vi "LogInfo2txt.vi"(7 "File ID":string, 11 "text":string) -> ()   [LabVIEW 2023, in "LoggingProber.lvlib"]
uses:
  LoggingProber.lvlib
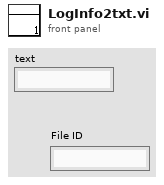
[diagram p1: front panel]
types:
  T1 = enum16{"open", "replace", "create", "open or create", "replace or create", "replace or create with confirmation"}
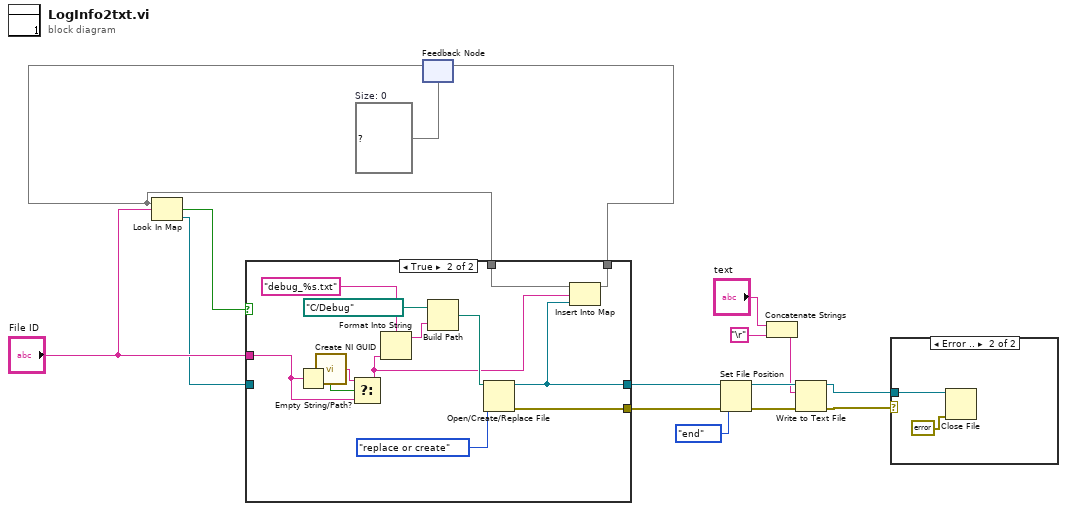
[diagram p0: block diagram]
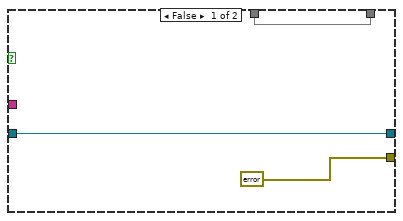
[diagram p2: hidden frame]
diagram:
  w1 = map{string, refnum<file>} {}  # Size: 0
  n1 = feedback #1(w1) -> (w4:map{string, refnum<file>})
  n2 = Look In Map(map=w4, key="File ID") -> (key not found?=w3:bool, value=w2:refnum<file>)  [unwired: 1 in]
  n3 = case shown="True" w3 {
    tunnel: [w19 w21] -> w6
    tunnel: [errorcluster {"status"=FALSE, "code"=0, "source"=""} ("error out") w32] -> w12
    tunnel: w2 -> [w19 _]
    tunnel: "File ID" -> [_ w24]
    tunnel: w4 -> [w17 w23]
    tunnel: [w17 w20] -> w5
    frame False {
    }
    frame True {
      n4 = Empty String/Path?(string/path=w24) -> (empty?=w26:bool)
      n5 = call <vilib>:"Create NI GUID.vi"() -> ("NI GUID"=w25:string)
      n6 = Select(t=w25, s=w26, f=w24) -> (s? t:f=w22:string)
      n7 = Format Into String(format string="debug_%s.txt", w22) -> (resulting string=w28:string)  [unwired: 2 in, 1 out]
      n8 = Build Path(base path=path "C:/Debug" ("file path (use dialog)"), name or relative path=w28) -> (appended path=w30:path)
      n9 = Open/Create/Replace File(file path (use dialog)=w30, operation (0:open)=T1."replace or create") -> (refnum out=w21:refnum<file>, error out=w32:errorcluster)  [unwired: 4 in, 1 out]
      n10 = Insert Into Map(map in=w23, key=w22, value=w21) -> (map out=w20:map{string, refnum<file>})  [unwired: 2 out]
    }
  }
  n11 = feedback-in #1(w5) -> ()
  n12 = Set File Position(refnum=w6, from (0:start)=enum16{"start", "end", "current"}."end", error in=w12) -> (refnum out=w13:refnum<file>, error out=w11:errorcluster)  [unwired: 1 in]
  n13 = Concatenate Strings("text", "\r") -> (w8:string)
  n14 = Write to Text File(file (use dialog)=w13, text=w8, error in=w11) -> (refnum out=w15:refnum<file>, error out=w16:errorcluster)  [unwired: 1 in, 1 out]
  n15 = case shown="Error .." w16 {
    tunnel: w15 -> [_ w33]
    frame No Error {
    }
    frame Error {
      n16 = Close File(refnum=w33, error in=errorcluster {"status"=FALSE, "code"=0, "source"=""}) -> ()  [unwired: 2 out]
    }
  }
